vi "RFSG Generate Pulse.vi"(7 "quantum":i32=4, 9 "IQ Rate (S/s)":dbl=10000000.0 format="%#.3p", 10 "Pulse Width (s)":dbl=0.0002 format="%#_6p", 11 "Pulse Repetition Interval [PRI] (s)":dbl=0.0009 format="%#_6p") -> (3 "IQ - Single Pulse":cdb[](array[numeric]))   [LabVIEW 2023]
panel:
  out "IQ - Single Pulse":dbl[](graph)
  out "size(s) 2":i32
  out "size(s)":i32
  out "IQ - Off":cdb[](array[numeric])
  out "IQ - On":cdb[](array[numeric])
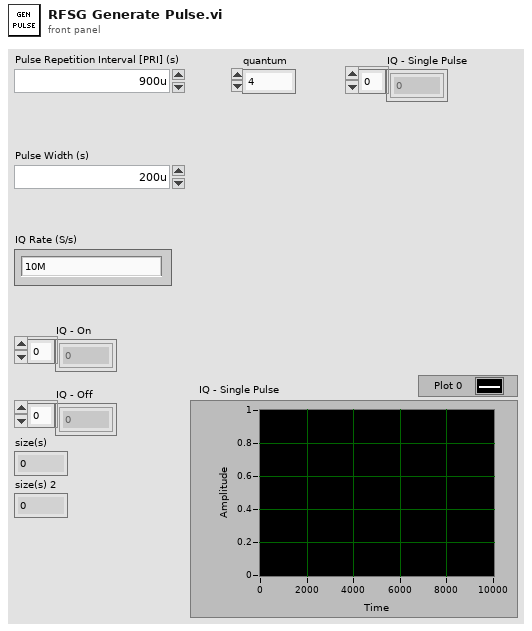
[diagram p1: front panel]
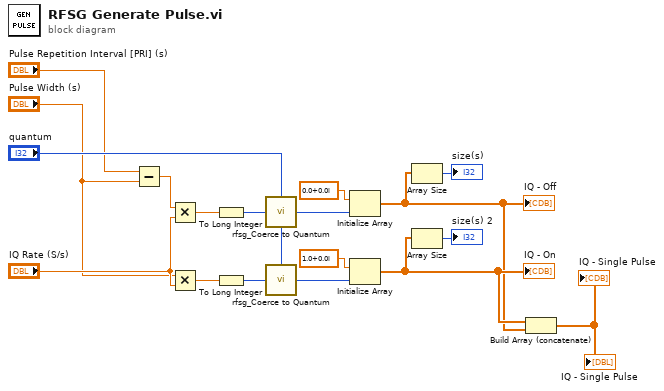
[diagram p0: block diagram]
diagram:
  n1 = Subtract(x="Pulse Repetition Interval [PRI] (s)", y="Pulse Width (s)") -> (x-y=w18:dbl)
  n2 = Multiply(x=w18, y="IQ Rate (S/s)") -> (x*y=w16:dbl)
  n3 = Multiply(x="Pulse Width (s)", y="IQ Rate (S/s)") -> (x*y=w13:dbl)
  n4 = To Long Integer(number=w16) -> (32bit integer=w10:i32)
  n5 = To Long Integer(number=w13) -> (32bit integer=w12:i32)
  n6 = call <instrlib>:"rfsg_Coerce to Quantum.vi"("quantum"="quantum", "samples"=w10) -> ("coerced to quantum"=w9:i32)  [unwired: 2 in]
  n7 = call <instrlib>:"rfsg_Coerce to Quantum.vi"("quantum"="quantum", "samples"=w12) -> ("coerced to quantum"=w11:i32)  [unwired: 2 in]
  n8 = Initialize Array(cdb 0.0+0.0i ("element"), w9) -> (w4:cdb[])
  "IQ - Off" <- w4
  n9 = Initialize Array(cdb 1.0+0.0i ("element"), w11) -> (w5:cdb[])
  "IQ - On" <- w5
  n10 = Array Size(array=w4) -> (size(s)=→"size(s)":i32)
  n11 = Array Size(array=w5) -> (size(s)=→"size(s) 2":i32)
  n12 = Build Array (concatenate)(w5, w4) -> (→"IQ - Single Pulse" →"IQ - Single Pulse":cdb[])
